vi "get_samples_in_directory.vi"(8 "Error In":errorcluster, 11 "Data Directory":path) -> (0 "Error Out":errorcluster, 3 "Samples":string[](array[string]))   [LabVIEW 2019]
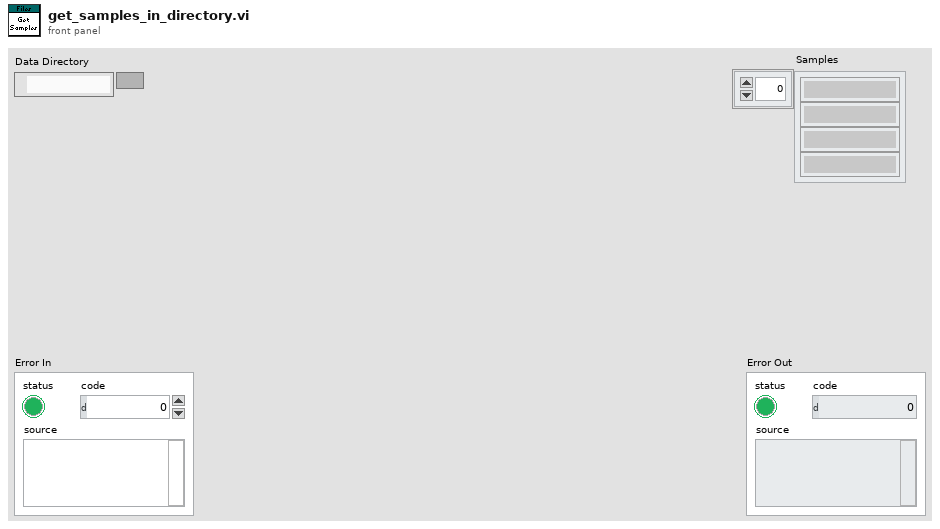
[diagram p1: front panel]
types:
  T1 = typedef "image_property_cluster_typedef.ctl" = cluster{"Stage Angle":dbl, "Sample Angle":dbl, "Polarizer 1 Angle":dbl, "Polarizer 2 Angle":dbl, "Sample Name":string}
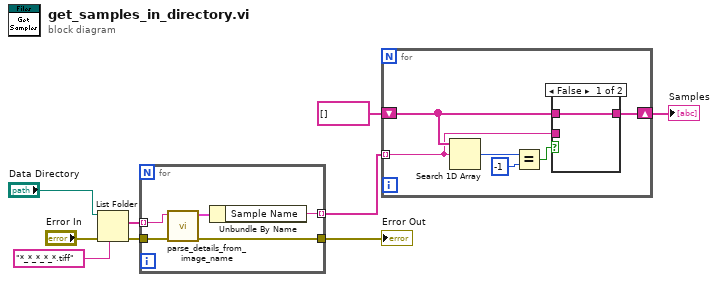
[diagram p0: block diagram]
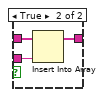
[diagram p2: hidden frame]
diagram:
  n1 = List Folder(path="Data Directory", pattern="*_*_*_*_*.tiff", error in="Error In") -> (filenames=w6:string[], error out=w2:errorcluster)  [unwired: 1 in, 2 out]
  n2 = for {
    tunnel: w6 -> [w14] mode=indexing
    tunnel: [w12] -> w5 mode=indexing
    tunnel: w2 -> [w11]
    tunnel: [w10] -> w1
    n3 = call "parse_details_from_image_name.vi"("Error In"=w11, "Image Name"=w14) -> ("Error Out"=w10:errorcluster, "Image Properties"=w13:T1)  [unwired: 8 in]
    n4 = Unbundle By Name(w13) -> ("Sample Name"=w12:string)
  }
  "Error Out" <- w1
  n5 = for {
    tunnel: w5 -> [w16] mode=indexing
    shift-right: [w15] -> w3
    shift-left: string[] [] -> [w18]
    n6 = Search 1D Array(1D array=w18, element=w16) -> (index of element=w20:i32)  [unwired: 1 in]
    n7 = Equal?(x=w20, y=-1) -> (x = y?=w17:bool)
    n8 = case shown="False" w17 {
      tunnel: w18 -> [w21 w24]
      tunnel: w16 -> [_ w23]
      tunnel: [w21 w22] -> w15
      frame False {
      }
      frame True {
        n9 = Insert Into Array(array=w24, new element=w23) -> (w22:string[])  [unwired: 1 in]
      }
    }
  }
  "Samples" <- w3
